vi "Main.vi"(8 "error in (no error)":errorcluster, 11 "ThorcamBase in":refnum<class "Thorcam.lvclass">) -> (0 "error out":errorcluster, 3 "conponent":refnum<class "Thorcam.lvclass">)   [LabVIEW 2012, in "Thorcam.lvclass"]
doc: "Main VI of the component."
uses:
  Thorcam.lvclass
  <vilib>/Distrio/Murmex/Murmex/command_enum.ctl
  feed.ctl
  current task.ctl
  Thorcam.lvclass/Thorcam.ctl
  <vilib>/Distrio/Murmex/InitialiseMessage/InitialiseMessage.lvclass
  <vilib>/Distrio/Murmex/Murmex/update_cluster.ctl
  <vilib>/Distrio/Murmex/GenericMessage/GenericMessage.lvclass
  <vilib>/Distrio/Murmex/ResetMessage/ResetMessage.lvclass
  <vilib>/Distrio/Murmex/StartMessage/run mode enum.ctl
  <vilib>/Distrio/Murmex/StopMessage/StopMessage.lvclass
  <vilib>/Distrio/Murmex/StartMessage/StartMessage.lvclass
  <vilib>/Distrio/Murmex/ConfigureMessage/ConfigureMessage.lvclass
  <vilib>/Distrio/Murmex/TerminateMessage/TerminateMessage.lvclass
  <vilib>/Distrio/Murmex/Murmex/Set configure at initialise.vi
  <vilib>/Distrio/Murmex/Murmex/Set log reference.vi
  <vilib>/Distrio/Murmex/Murmex/Set VI reference.vi
  <vilib>/Distrio/Murmex/Murmex/Get ID.vi
  <vilib>/Distrio/Murmex/Murmex/Set write log to disk.vi
  <vilib>/Distrio/Murmex/Message/Add or replace parameter.vi
  <vilib>/Distrio/Murmex/Murmex/Murmex.lvclass
  <vilib>/Distrio/Murmex/Message/Message.lvclass
panel:
  in  "Pre Tomo":bool
  out "status":string
  out "z step":dbl[unit]
  out "z2":dbl[unit]
  out "z1":dbl[unit]
  out "y":dbl[unit]
  out "x":dbl[unit]
  in  "button:free run":bool
  in  "button:quit":bool
  in  "button:configure":bool
  out "terminate?":bool
  in  "Tab Control":T1(tab)
  in  "Feed":T2=enum."Cross Correlation"
  in  "Filename":string="trial"
  in  "holdET":bool caption="hold"
  in  "holdPC":bool caption="hold"
  out "Video":T3(plugin-control)
  out "max pixel clock":dbl[unit] caption="max"
  out "min pixel clock":dbl[unit] caption="min"
  in  "pixel clock":dbl[unit] min=5000000.0 max=43000000.0
  out "max frames per second":dbl caption="max"
  out "min frames per second":dbl caption="min"
  in  "frames per second":dbl min=1.0159826258843114 max=2.908759204768504 step=3121.0986267166045
  out "max exp time":dbl[unit] caption="max"
  out "min exp time":dbl[unit] caption="min"
  in  "exposure time":dbl[unit] min=0.00032040000000000004 max=0.0004998240000000001 step=0.00032040000000000004
  in  "hot pixel correction":bool
  in  "gain":dbl min=0.0 max=255.0 step=1.0
  out "offset":i32 min=0 max=255 step=1
  out "gamma":i32=1 min=1 max=1000 step=1
  in  "button:reset":bool
  in  "button:save_tiff":bool
  in  "Select AOI":bool
  out "current task":T4
  in  "button::send move":bool
  in  "button::set as focus":bool
  out "Crosscorrelation":T3(plugin-control)
  in  "Autofocus":bool
  in  "phase comparison threshold":dbl
  in  "phase comparison interval":dbl[unit]
  out "ROB":T3(plugin-control)
  out "ROY":T3(plugin-control)
  out "pixel shift":dbl
  out "alignment quality":dbl
  out "translation":dbl[unit]
  in  "Number of Frames":i32
  in  "button:single frame":bool
  in  "command":T5
  in  "generic command":string
  out "log":string
  in  "Component id":string="Thor"
  in  "button:send command":bool
  # "current stack"
  # "Saving options"
  # "image acquisition"
  # "image correction"
  # "exposure time"
  # "frames per second"
  # "pixel clock"
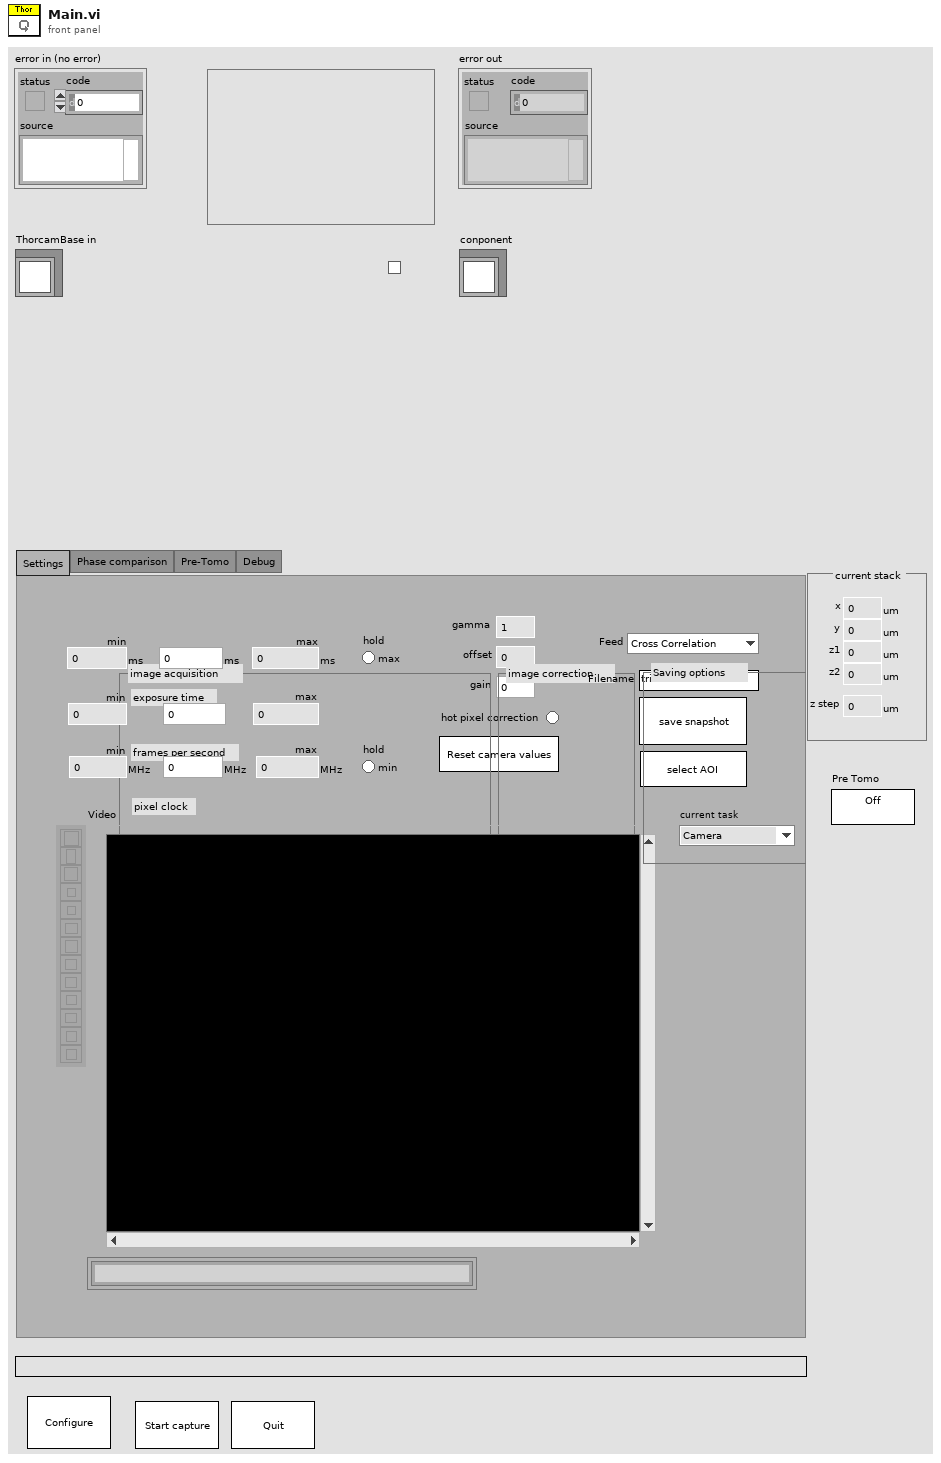
[diagram p1: front panel]
types:
  T1 = enum32{"Settings", "Phase comparison", "Pre-Tomo", "Debug"}
  T2 = typedef "Thorcam.lvclass/feed.ctl" = enum16{"Video", "Cross Correlation", "Rob and Roy", "Roy", "Rob"}
  T3 = typedef "IMAQ Image.ctl" = refnum<image>
  T4 = typedef "Thorcam.lvclass/current task.ctl" = enum16{"Camera", "Phase Comparison", "Pre-Tomo"}
  T5 = typedef "Murmex.lvlib/Murmex.lvclass/command_enum.ctl" = enum16{"null", "initialise", "reset", "terminate", "acknowledge", "update", "inspect", "inform", "proceed", "start", "stop", "fetch", "configure", "generic"}
  T6 = typedef "Murmex.lvlib/Murmex.lvclass/update_cluster.ctl" = cluster{"target ID":string, "key chains":string[], "values":variant[]}
  T7 = typedef "Murmex.lvlib/StartMessage.lvclass/run mode enum.ctl" = enum16{"infinite", "finite"}
  T8 = enum8{"Enabled", "Disabled", "Disabled and Grayed Out"}
  T9 = typedef "Murmex.lvclass/command_enum.ctl" = enum16{"null", "initialise", "reset", "terminate", "acknowledge", "update", "inspect", "inform", "proceed", "start", "stop", "fetch", "configure", "generic"}
  T10 = typedef "Murmex.lvclass/Event type enumerations.ctl" = enum16{"before", "after"}
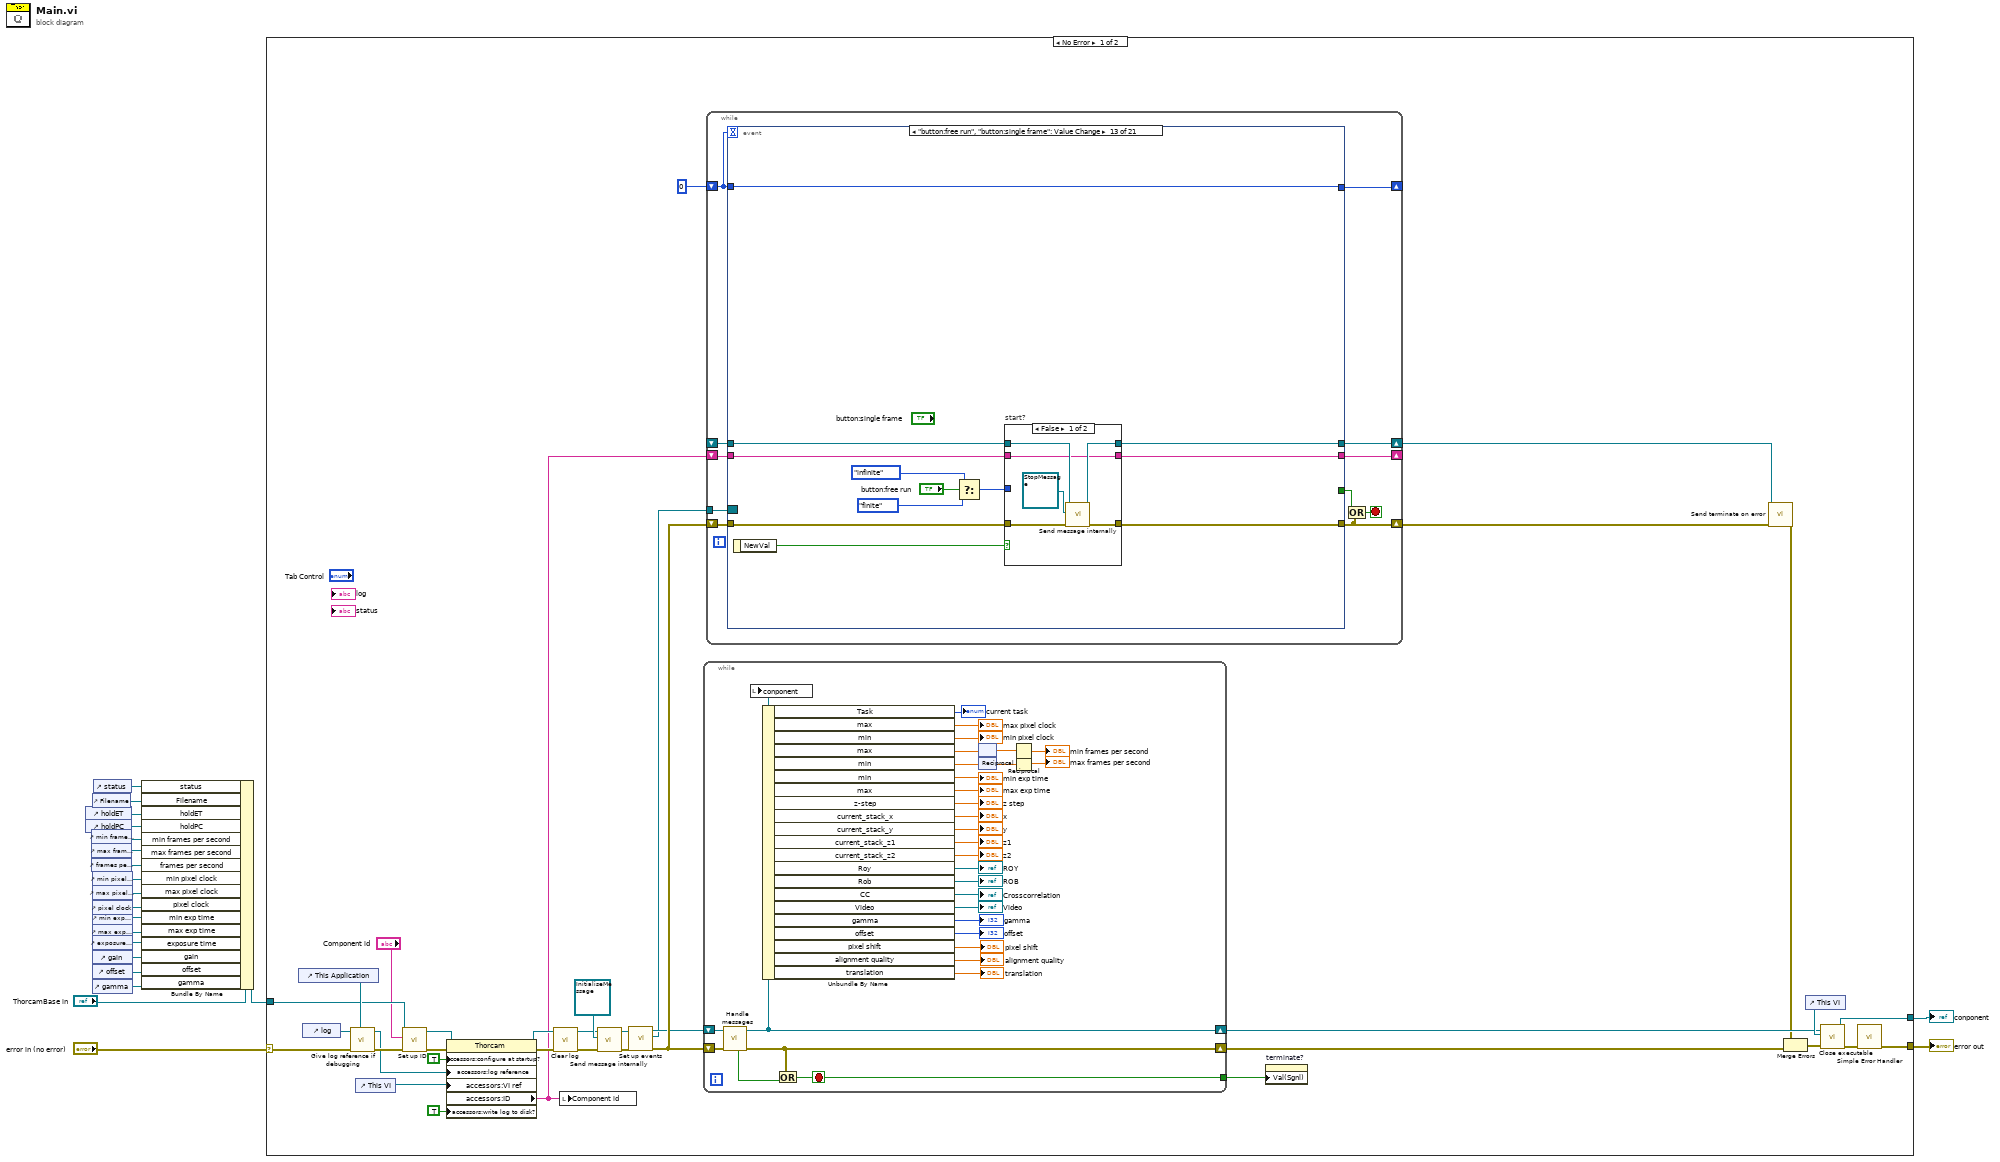
[diagram p0: block diagram]
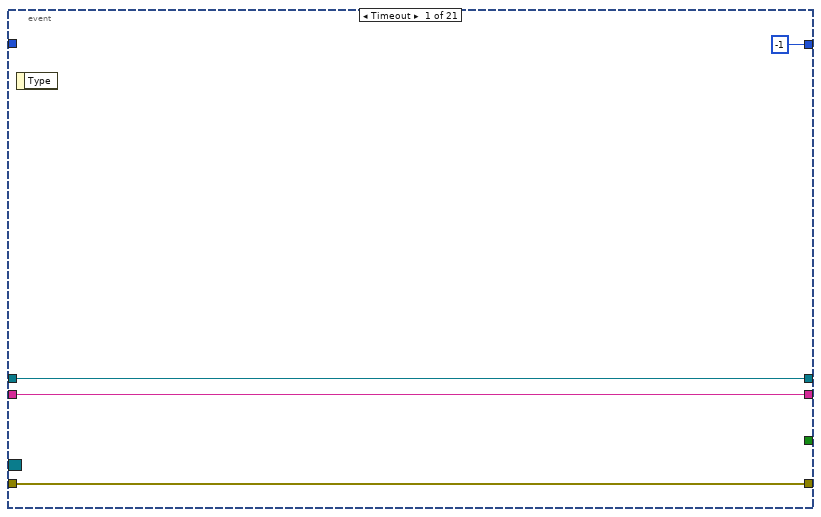
[diagram p2: hidden frame]
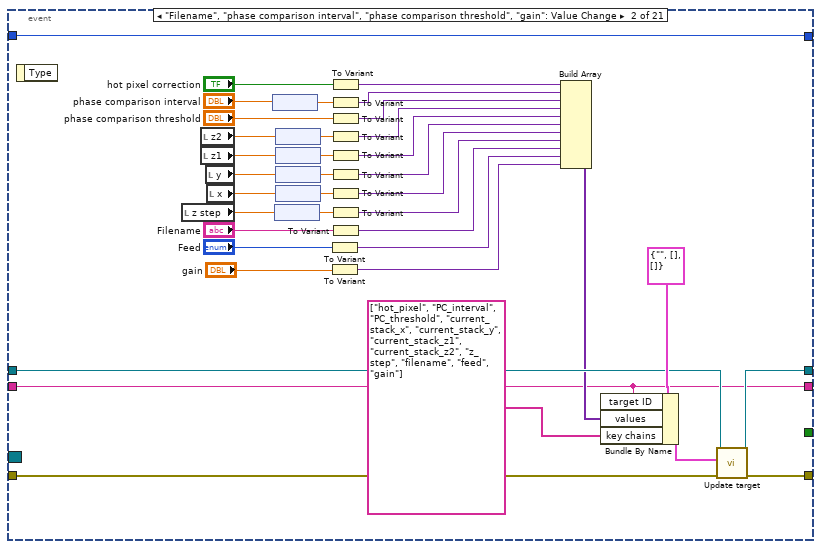
[diagram p3: hidden frame]
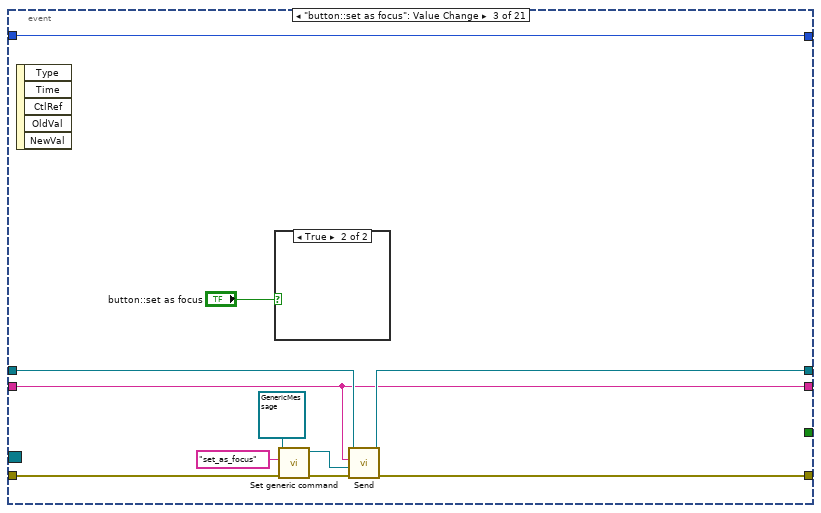
[diagram p4: hidden frame]
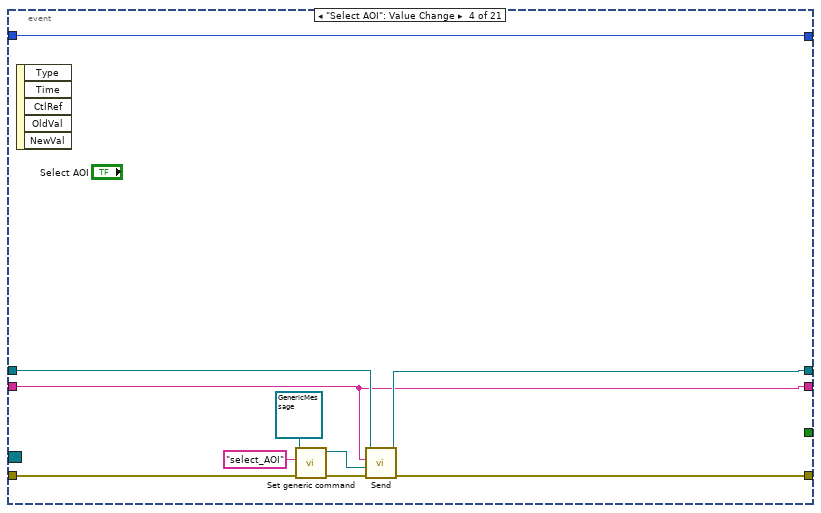
[diagram p6: hidden frame]
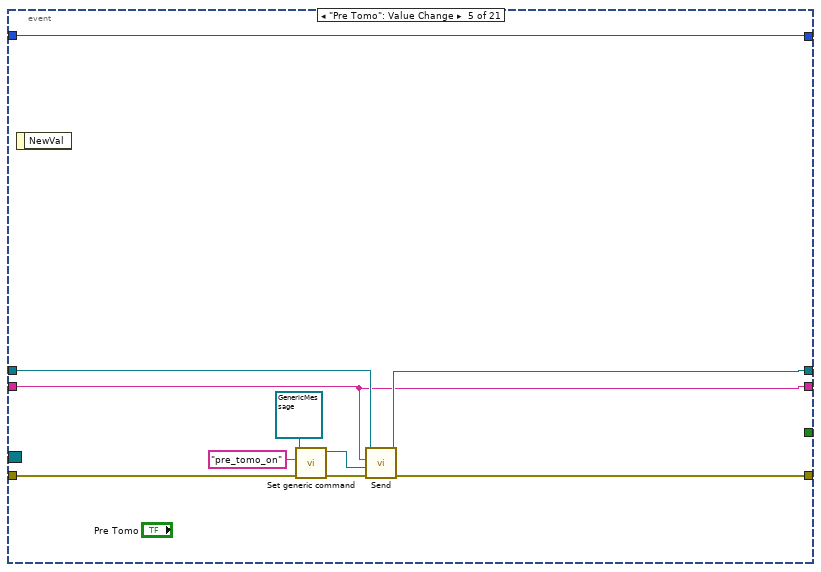
[diagram p7: hidden frame]
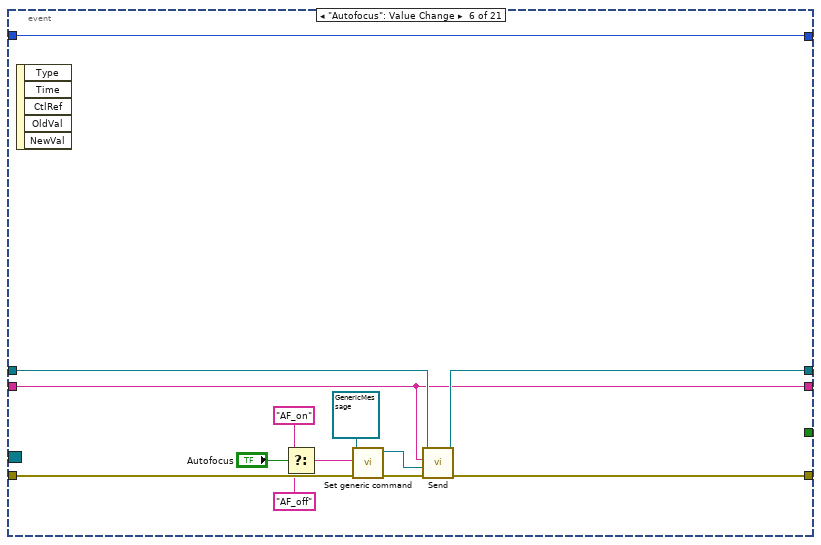
[diagram p8: hidden frame]
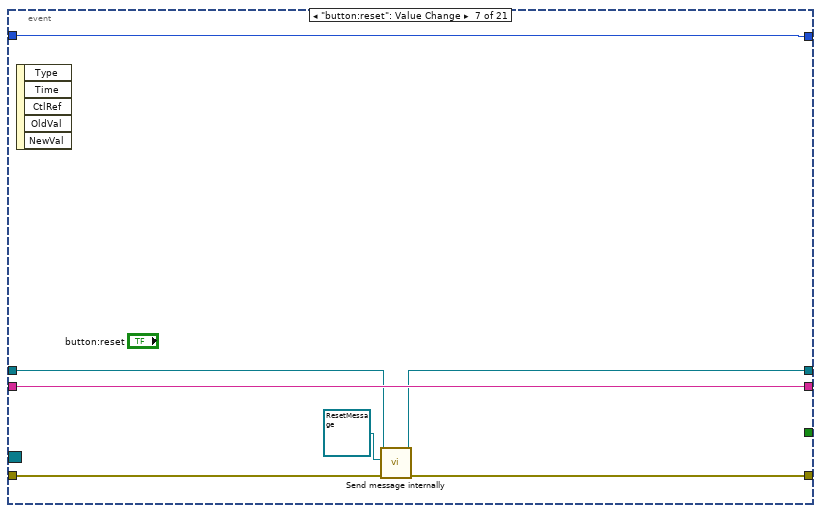
[diagram p9: hidden frame]
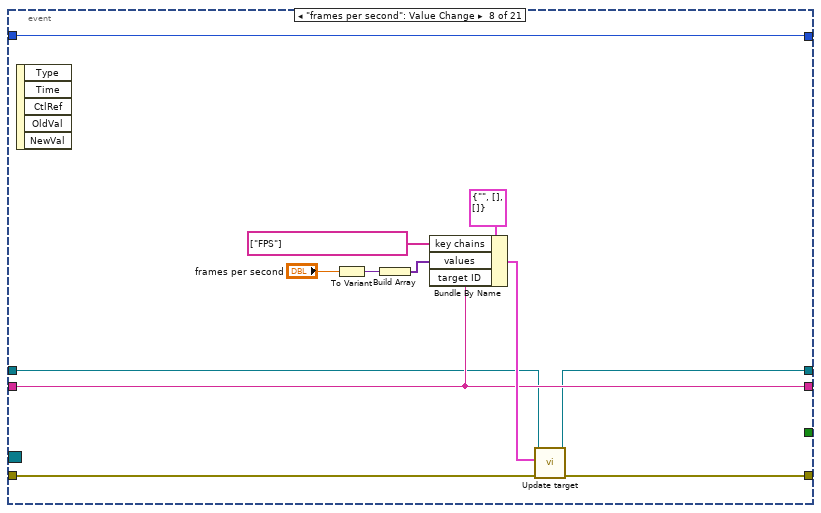
[diagram p10: hidden frame]
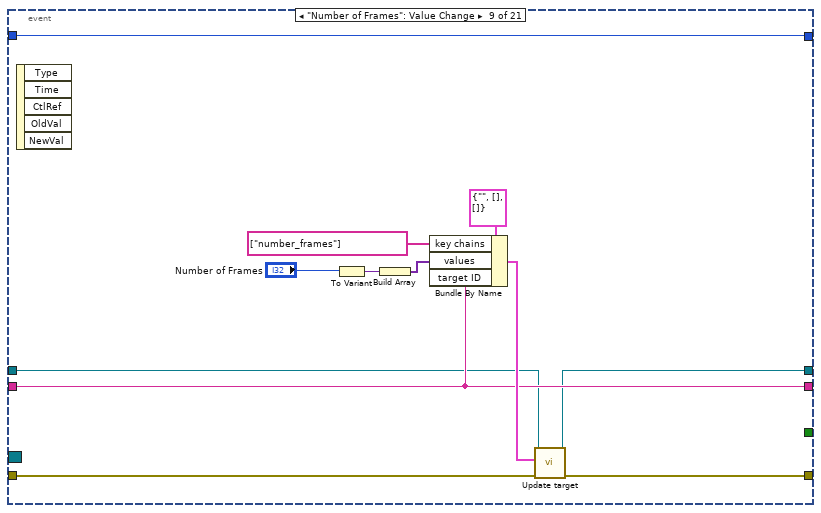
[diagram p11: hidden frame]
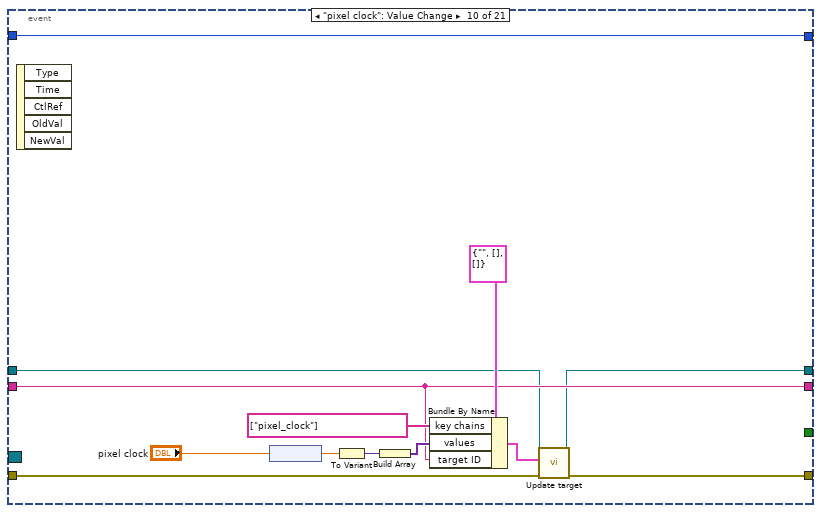
[diagram p12: hidden frame]
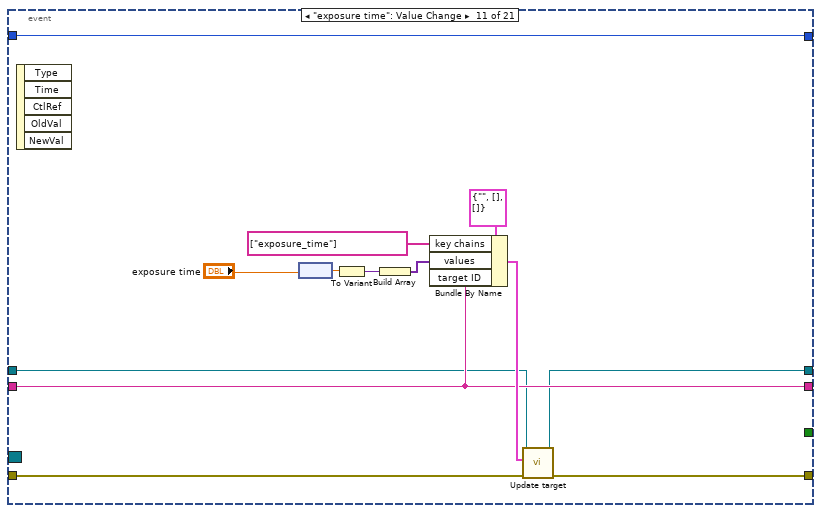
[diagram p13: hidden frame]
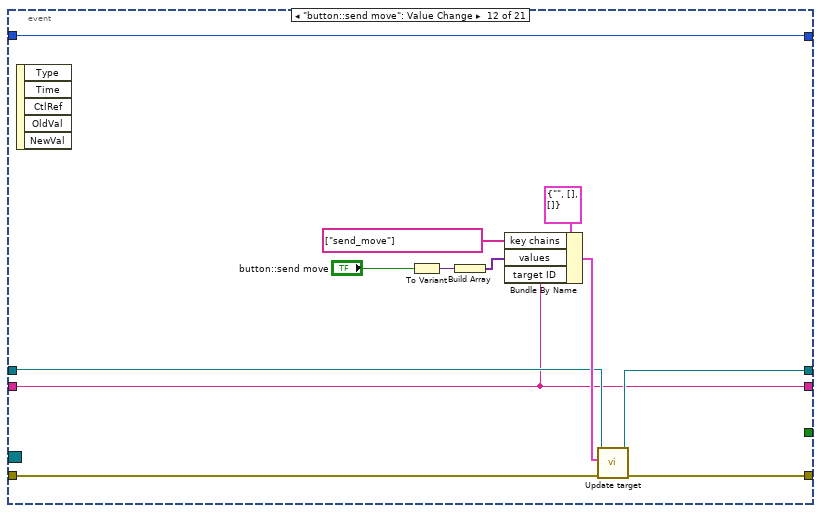
[diagram p14: hidden frame]
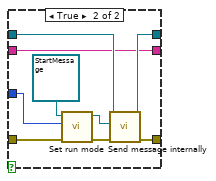
[diagram p15: hidden frame]
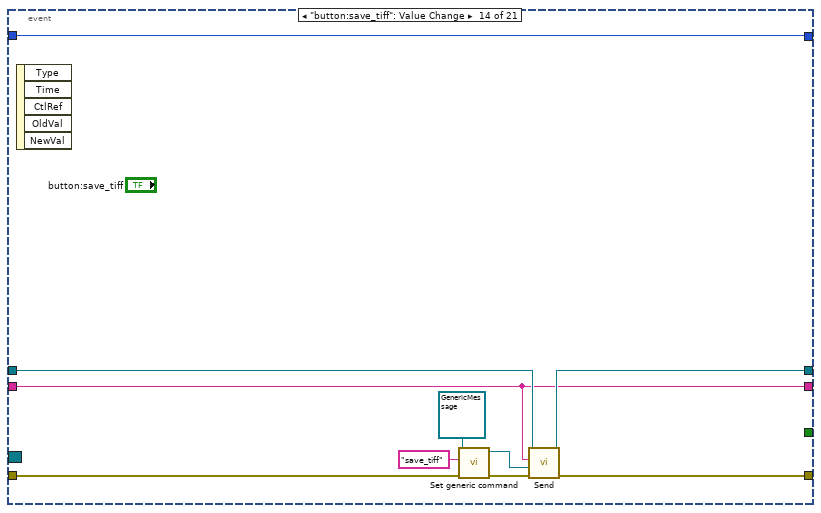
[diagram p16: hidden frame]
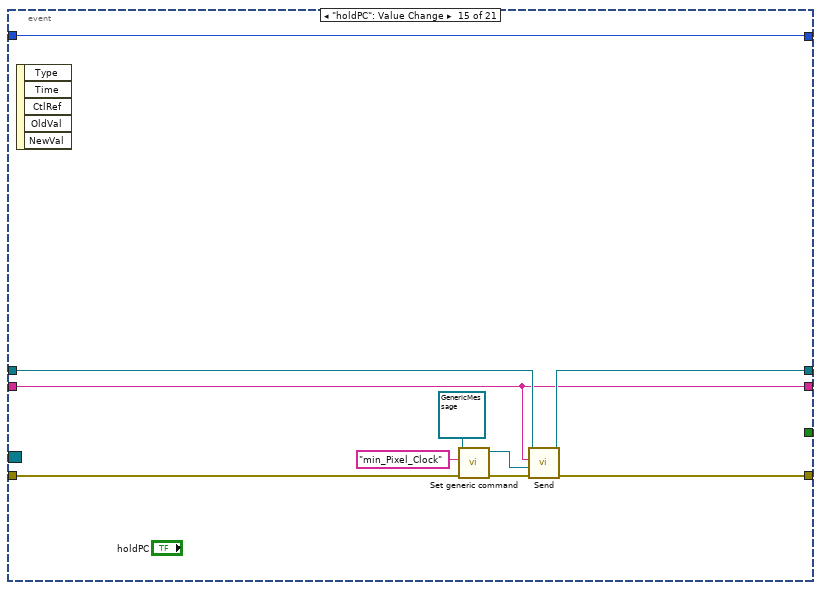
[diagram p17: hidden frame]
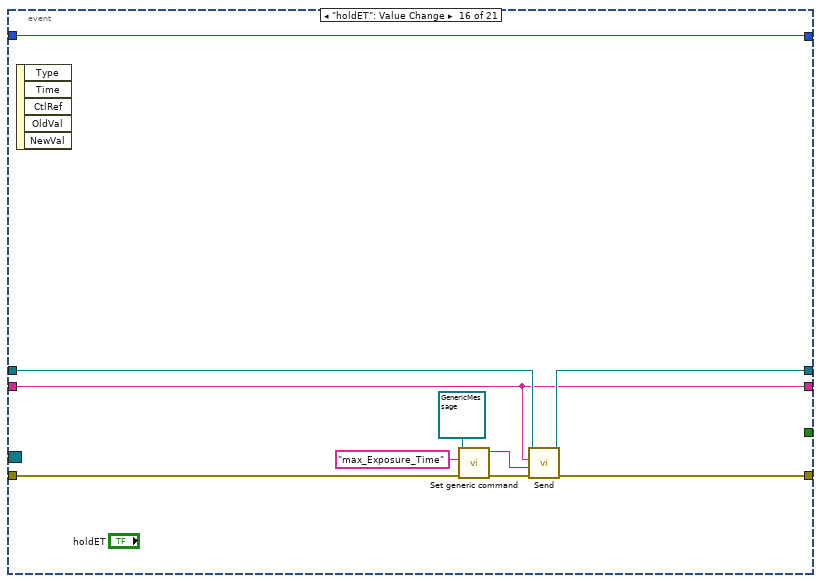
[diagram p18: hidden frame]
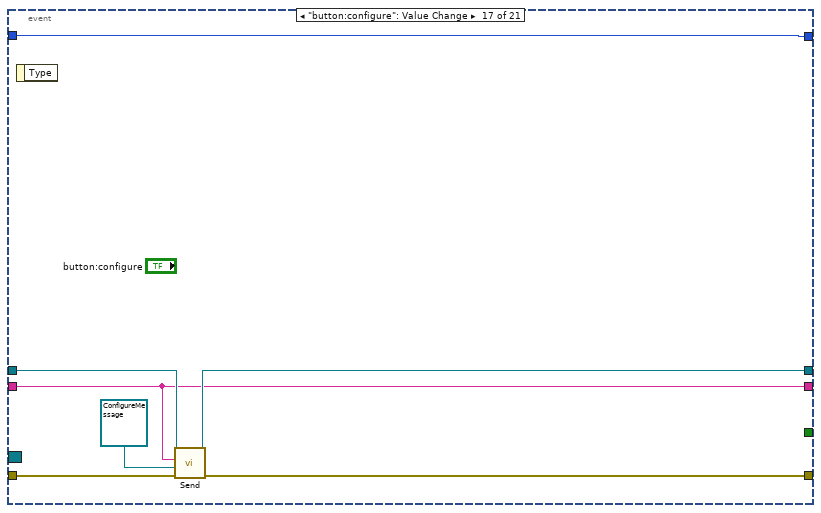
[diagram p19: hidden frame]
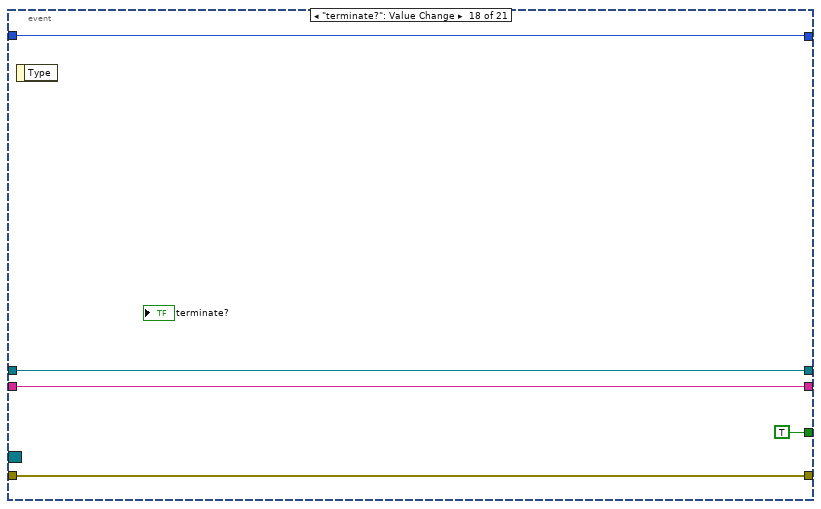
[diagram p20: hidden frame]
diagram:
  n1 = control-ref of="holdET"() -> (w3:refnum<vi>)
  n2 = control-ref of="holdPC"() -> (w4:refnum<vi>)
  n3 = control-ref of="min frames per second"() -> (w6:refnum<vi>)
  n4 = control-ref of="max frames per second"() -> (w5:refnum<vi>)
  n5 = control-ref of="frames per second"() -> (w7:refnum<vi>)
  n6 = control-ref of="min pixel clock"() -> (w8:refnum<vi>)
  n7 = control-ref of="max pixel clock"() -> (w9:refnum<vi>)
  n8 = control-ref of="pixel clock"() -> (w10:refnum<vi>)
  n9 = control-ref of="min exp time"() -> (w11:refnum<vi>)
  n10 = control-ref of="max exp time"() -> (w12:refnum<vi>)
  n11 = control-ref of="exposure time"() -> (w13:refnum<vi>)
  n12 = control-ref of="gain"() -> (w14:refnum<vi>)
  n13 = control-ref of="offset"() -> (w16:refnum<vi>)
  n14 = control-ref of="gamma"() -> (w15:refnum<vi>)
  n15 = control-ref of="Filename"() -> (w2:refnum<vi>)
  n16 = control-ref of="status"() -> (w1:refnum<vi>)
  n17 = Bundle By Name(cluster="ThorcamBase in", "status"=w1, "Filename"=w2, "holdET"=w3, "holdPC"=w4, "min frames per second"=w6, "max frames per second"=w5, "frames per second"=w7, "min pixel clock"=w8, "max pixel clock"=w9, "pixel clock"=w10, "min exp time"=w11, "max exp time"=w12, "exposure time"=w13, "gain"=w14, "offset"=w16, "gamma"=w15) -> (w17:refnum<class "Thorcam.lvclass">)
  n18 = case shown="No Error" "error in (no error)" {
    selector: "error in (no error)" -> [w54 w370]
    tunnel: w17 -> [w52 w369]
    tunnel: [w34 w370] -> w20
    tunnel: [w33 w369] -> w19
    frame No Error {
      n19 = control-ref of="This Application"() -> (w56:refnum<vi>)
      n20 = control-ref of="log"() -> (w55:refnum<vi>)
      n21 = call "Give log reference if debugging.vi"("application ref"=w56, "error in (no error)"=w54, "log reference in"=w55) -> ("error out"=w53:errorcluster, "log reference out"=w48:refnum<vi>)  [unwired: 6 in, 1 out]
      n22 = control-ref of="This VI"() -> (w47:refnum<vi>)
      n23 = call <vilib>:"Set up ID.vi"("error in (no error)"=w53, "component ID"="Component id", "MurmexBase in"=w52) -> ("error out"=w51:errorcluster, "MurmexBase out"=w50:refnum<class "Thorcam.lvclass">)  [unwired: 6 in, 1 out]
      n24 = property class="Thorcam"(reference=w50, error in=w51, "accessors:configure at startup?"=TRUE ("configure at startup?"), "accessors:log reference"=w48, "accessors:VI ref"=w47, "accessors:write log to disk?"=TRUE ("write log to disk?")) -> (reference out=w40:refnum<class "Thorcam.lvclass">, error out=w41:errorcluster, "accessors:ID"=w26:string)
      n25 = call <vilib>:"Clear log.vi"("error in (no error)"=w41, "MurmexBase in"=w40) -> ("error out"=w43:errorcluster, "MurmexBase out"=w42:refnum<class "Thorcam.lvclass">)  [unwired: 8 in]
      n26 = local write "Component id"(w26) -> ()
      n27 = call <vilib>:"Send message internally.vi"("error in (no error)"=w43, "Message"=refnum<class "InitialiseMessage.lvclass"> refnum ("InitialiseMessage"), "Murmex in"=w42) -> ("error out"=w45:errorcluster, "Murmex out"=w46:refnum<class "Thorcam.lvclass">)  [unwired: 7 in]
      n28 = call <vilib>:"Set up events.vi"("error in (no error)"=w45, "MurmexBase in"=w46) -> ("error out"=w39:errorcluster, "Event Registration Refnum"=w25:refnum<event-registration>, "MurmexBase out"=w38:refnum<class "Thorcam.lvclass">)  [unwired: 7 in]
      n29 = while {
        shift-right: [w365] -> w31
        shift-left: w39 -> [w368]
        shift-right: [w363] -> w32
        shift-left: w38 -> [w367]
        tunnel: [w364] -> w28
        stop <- w364 stop-if-true
        n30 = call <vilib>:"Handle messages.vi"("error in (no error)"=w368, "Murmex in"=w367) -> ("error out"=w365:errorcluster, "Murmex out"=w363:refnum<class "Thorcam.lvclass">, "terminated?"=w366:bool)  [unwired: 7 in]
        n31 = local write "conponent"(w363) -> ()
        n32 = Unbundle By Name(w363) -> ("Task"=→"current task":T4, "max"=→"max pixel clock":dbl[unit], "min"=→"min pixel clock":dbl[unit], "max"=w351:dbl[unit], "min"=w348:dbl[unit], "min"=→"min exp time":dbl[unit], "max"=→"max exp time":dbl[unit], "z-step"=→"z step":dbl[unit], "current_stack_x"=→"x":dbl[unit], "current_stack_y"=→"y":dbl[unit], "current_stack_z1"=→"z1":dbl[unit], "current_stack_z2"=→"z2":dbl[unit], "Roy"=→"ROY":T3, "Rob"=→"ROB":T3, "CC"=→"Crosscorrelation":T3, "Video"=→"Video":T3, "gamma"=→"gamma":i32, "offset"=→"offset":i32, "pixel shift"=→"pixel shift":dbl, "alignment quality"=→"alignment quality":dbl, "translation"=→"translation":dbl[unit])
        n33 = Or(x=w365, y=w366) -> (x .or. y?=w364:bool)
        n34 = node(w351) -> (w350:dbl)
        n35 = node(w348) -> (w347:dbl)
        n36 = Reciprocal(x=w350) -> (1/x=→"min frames per second":dbl)
        n37 = Reciprocal(x=w347) -> (1/x=→"max frames per second":dbl)
      }
      n38 = while {
        shift-right: [w60] -> w30
        shift-left: w39 -> [w66]
        shift-right: [w67] -> _
        shift-left: 0 -> [w57]
        shift-right: [w64] -> _
        shift-left: w26 -> [w65]
        tunnel: w25 -> [w63]
        shift-right: [w62] -> w24
        shift-left: _ -> [w61]
        stop <- w59 stop-if-true
        n39 = event shown="[12] \"button:free run\", \"button:single frame\": Value Change" {
          selector: w63 -> [_ _ _ _ _ _ _ _ _ _ _ _ _ _ _ _ _ _ _ _ _]
          dyn-events: _ -> [_ _ _ _ _ _ _ _ _ _ _ _ _ _ _ _ _ _ _ _ _]
          timeout: w57 -> [_ _ _ _ _ _ _ _ _ _ _ _ _ _ _ _ _ _ _ _ _]
          tunnel: w57 -> [_ w104 w111 w121 w131 w146 w159 w166 w178 w191 w204 w212 w232 w250 w260 w270 w280 w290 w298 w299 w309]
          tunnel: [-1 w104 w111 w121 w131 w146 w159 w166 w178 w191 w204 w212 w232 w250 w260 w270 w280 w290 w298 w299 w309] -> w67
          tunnel: [w70 w107 w115 w125 w135 w149 w157 w169 w181 w194 w207 w216 w233 w254 w264 w274 w284 w289 w296 w303 w316] -> w60
          tunnel: w66 -> [w70 w103 w116 w126 w136 w150 w158 w167 w179 w192 w205 w217 w234 w255 w265 w275 w285 w289 w297 w304 w317]
          tunnel: w65 -> [w69 w99 w110 w122 w132 w141 w160 w164 w176 w189 w202 w211 w227 w251 w261 w271 w281 w287 w292 w302 w315]
          tunnel: [w69 w99 w110 w122 w132 w141 w160 w164 w176 w189 w202 w211 w226 w251 w261 w271 w281 w287 w292 w302 w314] -> w64
          tunnel: [w68 w106 w113 w123 w133 w147 w155 w162 w174 w186 w200 w214 w230 w252 w262 w272 w282 w288 w294 w300 w311] -> w62
          tunnel: w61 -> [w68 w105 w114 w124 w134 w148 w156 w163 w175 w187 w199 w215 w231 w253 w263 w273 w283 w288 w295 w301 w310]
          tunnel: [_ _ _ _ _ _ _ _ _ _ _ _ _ _ _ _ _ TRUE _ _ _] -> w58
          event Timeout {
            n40 = event-data() -> ()  [unwired: 1 in, 1 out]
          }
          event "Filename", "phase comparison interval", "phase comparison threshold", "gain": Value Change {
            n41 = event-data() -> ()  [unwired: 1 in, 1 out]
            n42 = local read "z step"() -> (w86:dbl[unit])
            n43 = local read "z2"() -> (w94:dbl[unit])
            n44 = local read "z1"() -> (w93:dbl[unit])
            n45 = local read "y"() -> (w92:dbl[unit])
            n46 = local read "x"() -> (w91:dbl[unit])
            n47 = node("phase comparison interval") -> (w80:dbl)
            n48 = node(w86) -> (w78:dbl)
            n49 = node(w94) -> (w84:dbl)
            n50 = node(w93) -> (w83:dbl)
            n51 = node(w92) -> (w82:dbl)
            n52 = node(w91) -> (w81:dbl)
            n53 = To Variant(anything="Feed") -> (Variant=w74:variant)
            n54 = To Variant(anything="gain") -> (Variant=w72:variant)
            n55 = To Variant(anything="hot pixel correction") -> (Variant=w101:variant)
            n56 = To Variant(anything=w80) -> (Variant=w96:variant)
            n57 = To Variant(anything="phase comparison threshold") -> (Variant=w95:variant)
            n58 = To Variant(anything=w84) -> (Variant=w90:variant)
            n59 = To Variant(anything=w83) -> (Variant=w89:variant)
            n60 = To Variant(anything=w82) -> (Variant=w88:variant)
            n61 = To Variant(anything=w81) -> (Variant=w87:variant)
            n62 = To Variant(anything=w78) -> (Variant=w85:variant)
            n63 = To Variant(anything="Filename") -> (Variant=w76:variant)
            n64 = Build Array(w101, w96, w95, w90, w89, w88, w87, w85, w76, w74, w72) -> (w100:variant[])
            n65 = Bundle By Name(cluster=T6 {"target ID"="", "key chains"=[], "values"=[]} ("update cluster"), "target ID"=w99, "values"=w100, "key chains"=string[] ["hot_pixel", "PC_interval", "PC_threshold", "current_stack_x", "current_stack_y", "current_stack_z1", "current_stack_z2", "z_step", "filename", "feed", "gain"]) -> (w109:T6)
            n66 = call <vilib>:"Update target.vi"("error in (no error)"=w103, "update cluster"=w109, "MurmexBase in"=w105) -> ("error out"=w107:errorcluster, "MurmexBase out"=w106:refnum<class "Murmex.lvclass">)  [unwired: 7 in]
          }
          event "button::set as focus": Value Change {
            n67 = event-data() -> ()  [unwired: 1 in, 5 out]
            n68 = case shown="True" "button::set as focus" {
              frame False {
              }
              frame True {
              }
            }
            n69 = call <vilib>:"Set generic command.vi"("error in (no error)"=w116, "generic command"="set_as_focus", "GenericMessage in"=refnum<class "GenericMessage.lvclass"> refnum ("Distrio Murmex 1.1:GenericMessage")) -> ("error out"=w118:errorcluster, "GenericMessage out"=w117:refnum<class "GenericMessage.lvclass">)  [unwired: 7 in]
            n70 = call <vilib>:"Send.vi"("error in (no error)"=w118, "Message"=w117, "recipient"=w110, "Murmex in"=w114) -> ("error out"=w115:errorcluster, "Murmex out"=w113:refnum<class "Murmex.lvclass">)  [unwired: 6 in]
          }
          event "Select AOI": Value Change {
            n71 = event-data() -> ()  [unwired: 1 in, 5 out]
            n72 = call <vilib>:"Set generic command.vi"("error in (no error)"=w126, "generic command"="select_AOI", "GenericMessage in"=refnum<class "GenericMessage.lvclass"> refnum ("Distrio Murmex 1.1:GenericMessage")) -> ("error out"=w128:errorcluster, "GenericMessage out"=w127:refnum<class "GenericMessage.lvclass">)  [unwired: 7 in]
            n73 = call <vilib>:"Send.vi"("error in (no error)"=w128, "Message"=w127, "recipient"=w122, "Murmex in"=w124) -> ("error out"=w125:errorcluster, "Murmex out"=w123:refnum<class "Murmex.lvclass">)  [unwired: 6 in]
          }
          event "Pre Tomo": Value Change {
            n74 = event-data() -> ()  [unwired: 1 in, 1 out]
            n75 = call <vilib>:"Set generic command.vi"("error in (no error)"=w136, "generic command"="pre_tomo_on", "GenericMessage in"=refnum<class "GenericMessage.lvclass"> refnum ("Distrio Murmex 1.1:GenericMessage")) -> ("error out"=w138:errorcluster, "GenericMessage out"=w137:refnum<class "GenericMessage.lvclass">)  [unwired: 7 in]
            n76 = call <vilib>:"Send.vi"("error in (no error)"=w138, "Message"=w137, "recipient"=w132, "Murmex in"=w134) -> ("error out"=w135:errorcluster, "Murmex out"=w133:refnum<class "Murmex.lvclass">)  [unwired: 6 in]
          }
          event "Autofocus": Value Change {
            n77 = event-data() -> ()  [unwired: 1 in, 5 out]
            n78 = Select(t="AF_on" ("generic command"), s="Autofocus", f="AF_off" ("generic command")) -> (s? t:f=w144:string)
            n79 = call <vilib>:"Set generic command.vi"("error in (no error)"=w150, "generic command"=w144, "GenericMessage in"=refnum<class "GenericMessage.lvclass"> refnum ("Distrio Murmex 1.1:GenericMessage")) -> ("error out"=w152:errorcluster, "GenericMessage out"=w151:refnum<class "GenericMessage.lvclass">)  [unwired: 7 in]
            n80 = call <vilib>:"Send.vi"("error in (no error)"=w152, "Message"=w151, "recipient"=w141, "Murmex in"=w148) -> ("error out"=w149:errorcluster, "Murmex out"=w147:refnum<class "Murmex.lvclass">)  [unwired: 6 in]
          }
          event "button:reset": Value Change {
            n81 = event-data() -> ()  [unwired: 1 in, 5 out]
            n82 = call <vilib>:"Send message internally.vi"("error in (no error)"=w158, "Message"=refnum<class "ResetMessage.lvclass"> refnum ("Message in"), "Murmex in"=w156) -> ("error out"=w157:errorcluster, "Murmex out"=w155:refnum<class "Murmex.lvclass">)  [unwired: 7 in]
          }
          event "frames per second": Value Change {
            n83 = event-data() -> ()  [unwired: 1 in, 5 out]
            n84 = To Variant(anything="frames per second") -> (Variant=w168:variant)
            n85 = Build Array(w168) -> (w165:variant[])
            n86 = Bundle By Name(cluster=T6 {"target ID"="", "key chains"=[], "values"=[]} ("update cluster"), "key chains"=string[] ["FPS"], "values"=w165, "target ID"=w164) -> (w171:T6)
            n87 = call <vilib>:"Update target.vi"("error in (no error)"=w167, "update cluster"=w171, "MurmexBase in"=w163) -> ("error out"=w169:errorcluster, "MurmexBase out"=w162:refnum<class "Murmex.lvclass">)  [unwired: 7 in]
          }
          event "Number of Frames": Value Change {
            n88 = event-data() -> ()  [unwired: 1 in, 5 out]
            n89 = To Variant(anything="Number of Frames") -> (Variant=w180:variant)
            n90 = Build Array(w180) -> (w177:variant[])
            n91 = Bundle By Name(cluster=T6 {"target ID"="", "key chains"=[], "values"=[]} ("update cluster"), "key chains"=string[] ["number_frames"], "values"=w177, "target ID"=w176) -> (w183:T6)
            n92 = call <vilib>:"Update target.vi"("error in (no error)"=w179, "update cluster"=w183, "MurmexBase in"=w175) -> ("error out"=w181:errorcluster, "MurmexBase out"=w174:refnum<class "Murmex.lvclass">)  [unwired: 7 in]
          }
          event "pixel clock": Value Change {
            n93 = event-data() -> ()  [unwired: 1 in, 5 out]
            n94 = node("pixel clock") -> (w188:dbl)
            n95 = To Variant(anything=w188) -> (Variant=w193:variant)
            n96 = Build Array(w193) -> (w190:variant[])
            n97 = Bundle By Name(cluster=T6 {"target ID"="", "key chains"=[], "values"=[]} ("update cluster"), "key chains"=string[] ["pixel_clock"], "values"=w190, "target ID"=w189) -> (w196:T6)
            n98 = call <vilib>:"Update target.vi"("error in (no error)"=w192, "update cluster"=w196, "MurmexBase in"=w187) -> ("error out"=w194:errorcluster, "MurmexBase out"=w186:refnum<class "Murmex.lvclass">)  [unwired: 7 in]
          }
          event "exposure time": Value Change {
            n99 = event-data() -> ()  [unwired: 1 in, 5 out]
            n100 = node("exposure time") -> (w201:dbl)
            n101 = To Variant(anything=w201) -> (Variant=w206:variant)
            n102 = Build Array(w206) -> (w203:variant[])
            n103 = Bundle By Name(cluster=T6 {"target ID"="", "key chains"=[], "values"=[]} ("update cluster"), "key chains"=string[] ["exposure_time"], "values"=w203, "target ID"=w202) -> (w209:T6)
            n104 = call <vilib>:"Update target.vi"("error in (no error)"=w205, "update cluster"=w209, "MurmexBase in"=w199) -> ("error out"=w207:errorcluster, "MurmexBase out"=w200:refnum<class "Murmex.lvclass">)  [unwired: 7 in]
          }
          event "button::send move": Value Change {
            n105 = event-data() -> ()  [unwired: 1 in, 5 out]
            n106 = To Variant(anything="button::send move") -> (Variant=w219:variant)
            n107 = Build Array(w219) -> (w218:variant[])
            n108 = Bundle By Name(cluster=T6 {"target ID"="", "key chains"=[], "values"=[]} ("update cluster"), "key chains"=string[] ["send_move"], "values"=w218, "target ID"=w211) -> (w221:T6)
            n109 = call <vilib>:"Update target.vi"("error in (no error)"=w217, "update cluster"=w221, "MurmexBase in"=w215) -> ("error out"=w216:errorcluster, "MurmexBase out"=w214:refnum<class "Murmex.lvclass">)  [unwired: 7 in]
          }
          event "button:free run", "button:single frame": Value Change {
            n110 = event-data() -> ("NewVal"=w228:bool)  [unwired: 1 in]
            n111 = Select(t=run_mode_enum."infinite" ("run mode"), s="button:free run", f=run_mode_enum."finite" ("run mode")) -> (s? t:f=w225:T7)
            n112 = case "start?" shown="False" w228 {
              tunnel: w234 -> [w240 w244]
              tunnel: [w239 w247] -> w233
              tunnel: w231 -> [w238 w249]
              tunnel: [w237 w248] -> w230
              tunnel: w227 -> [w236 w246]
              tunnel: [w236 w246] -> w226
              tunnel: w225 -> [_ w245]
              frame False {
                n113 = call <vilib>:"Send message internally.vi"("error in (no error)"=w240, "Message"=refnum<class "StopMessage.lvclass"> refnum ("Distrio Murmex 1.5:StopMessage"), "Murmex in"=w238) -> ("error out"=w239:errorcluster, "Murmex out"=w237:refnum<class "Murmex.lvclass">)  [unwired: 7 in]
              }
              frame True {
                n114 = call <vilib>:"Set run mode.vi"("error in (no error)"=w244, "run mode"=w245, "StartMessage in"=refnum<class "StartMessage.lvclass"> refnum ("Message in")) -> ("error out"=w243:errorcluster, "StartMessage out"=w241:refnum<class "StartMessage.lvclass">)  [unwired: 7 in]
                n115 = call <vilib>:"Send message internally.vi"("error in (no error)"=w243, "Message"=w241, "Murmex in"=w249) -> ("error out"=w247:errorcluster, "Murmex out"=w248:refnum<class "Murmex.lvclass">)  [unwired: 7 in]
              }
            }
          }
          event "button:save_tiff": Value Change {
            n116 = event-data() -> ()  [unwired: 1 in, 5 out]
            n117 = call <vilib>:"Set generic command.vi"("error in (no error)"=w255, "generic command"="save_tiff", "GenericMessage in"=refnum<class "GenericMessage.lvclass"> refnum ("Distrio Murmex 1.1:GenericMessage")) -> ("error out"=w257:errorcluster, "GenericMessage out"=w256:refnum<class "GenericMessage.lvclass">)  [unwired: 7 in]
            n118 = call <vilib>:"Send.vi"("error in (no error)"=w257, "Message"=w256, "recipient"=w251, "Murmex in"=w253) -> ("error out"=w254:errorcluster, "Murmex out"=w252:refnum<class "Murmex.lvclass">)  [unwired: 6 in]
          }
          event "holdPC": Value Change {
            n119 = event-data() -> ()  [unwired: 1 in, 5 out]
            n120 = call <vilib>:"Set generic command.vi"("error in (no error)"=w265, "generic command"="min_Pixel_Clock", "GenericMessage in"=refnum<class "GenericMessage.lvclass"> refnum ("Distrio Murmex 1.1:GenericMessage")) -> ("error out"=w267:errorcluster, "GenericMessage out"=w266:refnum<class "GenericMessage.lvclass">)  [unwired: 7 in]
            n121 = call <vilib>:"Send.vi"("error in (no error)"=w267, "Message"=w266, "recipient"=w261, "Murmex in"=w263) -> ("error out"=w264:errorcluster, "Murmex out"=w262:refnum<class "Murmex.lvclass">)  [unwired: 6 in]
          }
          event "holdET": Value Change {
            n122 = event-data() -> ()  [unwired: 1 in, 5 out]
            n123 = call <vilib>:"Set generic command.vi"("error in (no error)"=w275, "generic command"="max_Exposure_Time", "GenericMessage in"=refnum<class "GenericMessage.lvclass"> refnum ("Distrio Murmex 1.1:GenericMessage")) -> ("error out"=w277:errorcluster, "GenericMessage out"=w276:refnum<class "GenericMessage.lvclass">)  [unwired: 7 in]
            n124 = call <vilib>:"Send.vi"("error in (no error)"=w277, "Message"=w276, "recipient"=w271, "Murmex in"=w273) -> ("error out"=w274:errorcluster, "Murmex out"=w272:refnum<class "Murmex.lvclass">)  [unwired: 6 in]
          }
          event "button:configure": Value Change {
            n125 = event-data() -> ()  [unwired: 1 in, 1 out]
            n126 = call <vilib>:"Send.vi"("error in (no error)"=w285, "Message"=refnum<class "ConfigureMessage.lvclass"> refnum ("ConfigureMessage"), "recipient"=w281, "Murmex in"=w283) -> ("error out"=w284:errorcluster, "Murmex out"=w282:refnum<class "Murmex.lvclass">)  [unwired: 6 in]
          }
          event "terminate?": Value Change {
            n127 = event-data() -> ()  [unwired: 1 in, 1 out]
          }
          event "button:quit": Value Change {
            n128 = event-data() -> ()  [unwired: 1 in, 1 out]
            n129 = call <vilib>:"Send.vi"("error in (no error)"=w297, "Message"=refnum<class "TerminateMessage.lvclass"> refnum ("TerminateMessage"), "recipient"=w292, "Murmex in"=w295) -> ("error out"=w296:errorcluster, "Murmex out"=w294:refnum<class "Murmex.lvclass">)  [unwired: 6 in]
          }
          event "button:send command": Value Change {
            n130 = event-data() -> ()  [unwired: 1 in, 1 out]
            n131 = call <vilib>:"Create from command.vi"("error in (no error)"=w304, "generic command"="generic command", "command"="command") -> ("error out"=w308:errorcluster, "Message out"=w305:refnum<class "Message.lvclass">)  [unwired: 7 in]
            n132 = call <vilib>:"Send.vi"("error in (no error)"=w308, "Message"=w305, "recipient"=w302, "Murmex in"=w301) -> ("error out"=w303:errorcluster, "Murmex out"=w300:refnum<class "Murmex.lvclass">)  [unwired: 6 in]
          }
          event User Event {
            n133 = event-data() -> ("command"=w313:T9, "event type"=w312:T10)  [unwired: 1 in]
            n134 = case shown="\"null\", Default" w313 {
              tunnel: w312 -> [_ w327]
              tunnel: w317 -> [w318 w326]
              tunnel: w315 -> [w319 w325]
              tunnel: [w319 w324] -> w314
              tunnel: [w320 w323] -> w311
              tunnel: w310 -> [w320 w322]
              tunnel: [w318 w321] -> w316
              frame "null", Default {
              }
              frame "initialise" {
                n135 = case shown="\"after\"" w327 {
                  tunnel: w326 -> [w329 w337]
                  tunnel: [w328 w335] -> w321
                  tunnel: [w331 w334] -> w324
                  tunnel: w325 -> [w331 w334]
                  tunnel: [w332 w333] -> w323
                  tunnel: w322 -> [w332 _]
                  frame "before", Default {
                    n136 = property on="Tab Control" class="TabCtl (strict)"(error in=w329, "DisabledEnum"=T8."Disabled and Grayed Out" ("Disabled")) -> (error out=w328:errorcluster)  [unwired: 1 in, 1 out]
                  }
                  frame "after" {
                    n137 = local read "conponent"() -> (w333:refnum<class "Thorcam.lvclass">)
                    n138 = property on="Tab Control" class="TabCtl (strict)"(error in=w337, "DisabledEnum"=T8."Enabled" ("Disabled")) -> (error out=w335:errorcluster)  [unwired: 1 in, 1 out]
                  }
                }
              }
            }
          }
        }
        n139 = Or(x=w58, y=w60) -> (x .or. y?=w59:bool)
      }
      n140 = property on="terminate?" class="Bool (strict)"("Val(Sgnl)"=w28) -> ()  [unwired: 2 in, 2 out]
      n141 = call <vilib>:"Send terminate on error.vi"("error in (no error)"=w30, "Murmex in"=w24) -> ("error out"=w29:errorcluster)  [unwired: 8 in, 1 out]
      n142 = Merge Errors(w29, w31) -> (w36:errorcluster)
      n143 = control-ref of="This VI"() -> (w37:refnum<vi>)
      n144 = call <vilib>:"Close executable.vi"("error in (no error)"=w36, "main VI ref (optional)"=w37, "MurmexBase in"=w32) -> ("error out"=w35:errorcluster, "MurmexBase out"=w33:refnum<class "Thorcam.lvclass">)  [unwired: 7 in]
      n145 = call <vilib>:"Simple Error Handler.vi"("error in (no error)"=w35) -> ("error out"=w34:errorcluster)  [unwired: 4 in, 4 out]
    }
    frame Error {
    }
  }
  "error out" <- w20
  "conponent" <- w19
